vi "Pre Launch Init.vi"(11 "Blower in":refnum<class "Blower.lvclass">) -> (0 "error out":errorcluster, 3 "Blower out":refnum<class "Blower.lvclass">)   [LabVIEW 2015, in "cRIO-Carbondioxide.lvlib" / "CO2-Actor.lvlib" / "Blower.lvclass"]
doc: "(<B>Filename</B>: Actor Framework.lvlib:Actor.lvclass:Pre Launch Init.vi)\n\nDefines behavior that occurs after the Launch Actor method is invoked but before the actor's Actor Core method begins running.\n\nThe Pre Launch Init method is guaranteed to finish before the Launch Actor method returns to its caller and before the actor itself receives any messages. Any references that the Pre Launch Init method obtains are guaranteed to have the same lifetime as the actor itself. Any errors that the Pre Launch Init method returns will abort the launch.\n\nBy default, this method does nothing. A descendant class may override it to define behavior."
uses:
  Blower.lvclass
  Valve/Valve.lvclass
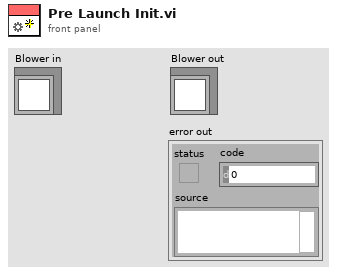
[diagram p1: front panel]
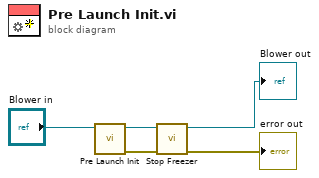
[diagram p0: block diagram]
diagram:
  n1 = call-parent "Pre Launch Init.vi"("Valve in"="Blower in") -> ("error out"=w4:errorcluster, "Valve out"=w3:refnum<class "Blower.lvclass">)  [unwired: 9 in]
  n2 = call "Stop Freezer.vi"("error in (no error)"=w4, "Blower in"=w3) -> ("error out"=→"error out":errorcluster, "Blower out"=→"Blower out":refnum<class "Blower.lvclass">)  [unwired: 8 in]
